vi "Read Ports_modified.vi"(0 "Refnum in":refnum<k20>, 2 "timeout (ms)":i32=5000, 5 "All 4 Ports":bool, 9 "number of elements":u64, 11 "error in":errorcluster, 13 "Simulated Data":bool) -> (4 "Refnum out":refnum<k20>, 6 "Read Region References":refnum<data-value>[](array[refnum]), 8 "Errors":u32[](array[numeric]), 10 "Elements Remaining":u32, 14 "Data Valid":bool, 15 "error out":errorcluster)   [LabVIEW 2016]
doc: "This VI wraps and calls the appropriate FIFO read node to access the FIFO corresponding to the input <b>port</b>\n\n<B>Input Parameters</B>\n\n<B>Refnum in</B> Receives a reference to the FPGA from the previous VI.\n\n<B>timeout (ms)</B> The timeout to pass to the FIFO read node\n\n<B>port</B> Selects which physical port to read from.\n\n<B>number of elements</B> Specifies the number of FIFO elements to read during this call.\n\n<B>error in</B> describes error conditions that occur before this node runs. This input provides standard error in functionality.\n\n<B>Output Parameters</B>\n\n<B>Refnum out</B> passes a reference to the FPGA to the next VI.\n\n<B>Receive Waveform</B> The data read from the device will be written to this output\n\n<B>Waveform Size</B> Indicates the number of samples in the output waveform\n\n<B>Elements Remaining</B> Indicates the number of samples presently waiting in the FIFO after the read.\n\n<B>error out</B> contains error information. This output provides standard error out functionality."
uses:
  Base Bitfile Reference.ctl
  <vilib>/Utility/error.llb/Error Cluster From Error Code.vi
  <vilib>/rvi/errors/niLvFpgaAdjustHostInterfaceError.vi
  <vilib>/rvi/interface/nirviMethod/nirviMethod.xnode
  <vilib>/rvi/interface/nirviReadWriteControl/nirviReadWriteControl.xnode
  Aurora Stream (NI 6592R) (Host).lvlib
  <vilib>/rvi/errors/niLvFpgaMergeErrorWithErrorCode.vi
  NiFpgaLv.dll
  <vilib>/rvi/interface/Simulation/niFpgaSimulationCallBeginRW.vi
  <vilib>/FPGAPlugInAG/Dynamic/niLvFpga_AcquireReadRegionFifo_Dynamic.vi
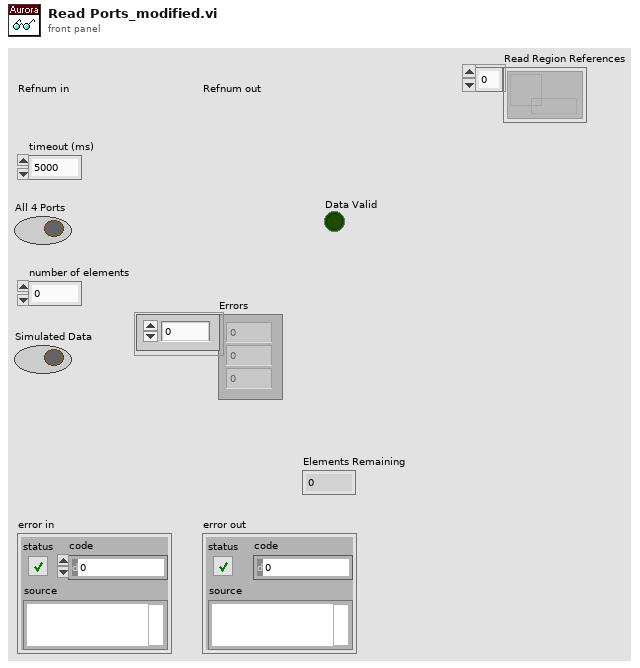
[diagram p1: front panel]
types:
  T1 = typedef "Aurora Stream (NI 6592R) (Host).lvlib/Base Bitfile Reference.ctl" = refnum<k20>
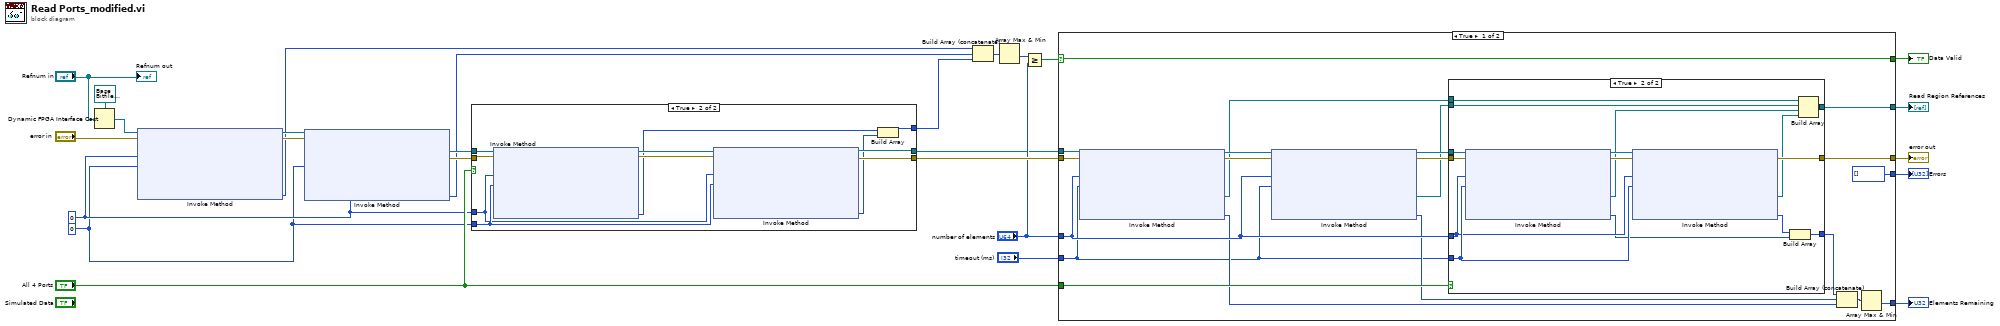
[diagram p0: block diagram]
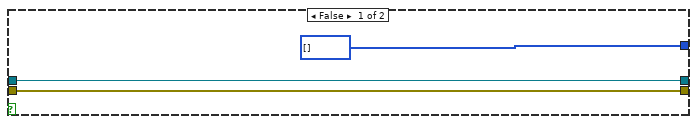
[diagram p2: hidden frame]
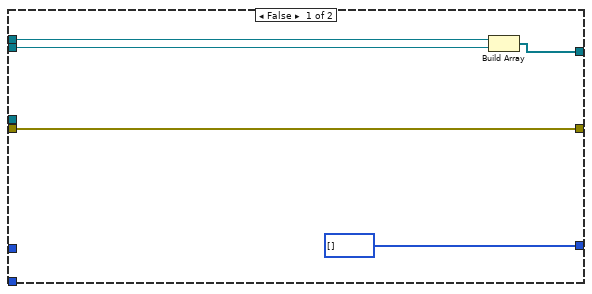
[diagram p3: hidden frame]
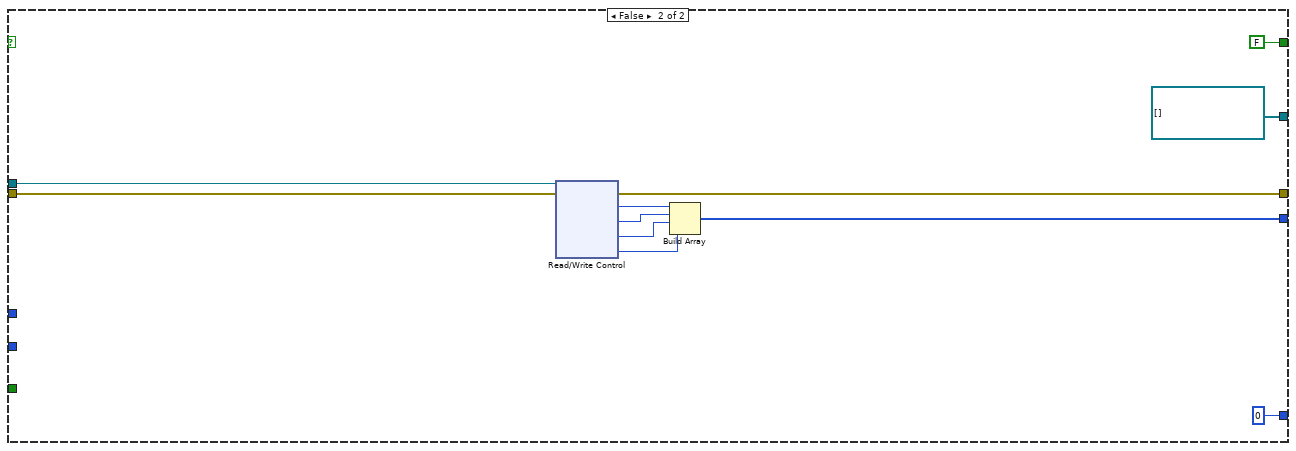
[diagram p4: hidden frame]
diagram:
  w5 = 0 ("Timeout (ms)")
  w6 = u32 0 ("Number of Elements")
  n1 = Dynamic FPGA Interface Cast(Session In=T1 refnum ("Aurora Sample Project"), Type="Refnum in") -> (Session Out=w13:T1)
  n2 = xnode "Invoke Method"("FPGA VI Reference In"=w13, "error in"="error in", "Number of Elements"=w6, "Timeout (ms)"=w5) -> ("FPGA VI Reference Out"=w11:T1, "error out"=w10:errorcluster, "Elements Remaining"=w2:u32)  [unwired: 2 out]
  n3 = xnode "Invoke Method"("FPGA VI Reference In"=w11, "error in"=w10, "Number of Elements"=w6, "Timeout (ms)"=w5) -> ("FPGA VI Reference Out"=w8:T1, "error out"=w9:errorcluster, "Elements Remaining"=w1:u32)  [unwired: 2 out]
  n4 = case shown="True" "All 4 Ports" {
    tunnel: w9 -> [w27 w38]
    tunnel: [w27 w35] -> w19
    tunnel: [u32[] [] w34] -> w22
    tunnel: w8 -> [w28 w37]
    tunnel: [w28 w36] -> w7
    tunnel: w6 -> [_ w30]
    tunnel: w5 -> [_ w31]
    frame False {
    }
    frame True {
      n5 = xnode "Invoke Method"("FPGA VI Reference In"=w37, "error in"=w38, "Number of Elements"=w30, "Timeout (ms)"=w31) -> ("FPGA VI Reference Out"=w39:T1, "error out"=w40:errorcluster, "Elements Remaining"=w33:u32)  [unwired: 2 out]
      n6 = xnode "Invoke Method"("FPGA VI Reference In"=w39, "error in"=w40, "Number of Elements"=w30, "Timeout (ms)"=w31) -> ("FPGA VI Reference Out"=w36:T1, "error out"=w35:errorcluster, "Elements Remaining"=w32:u32)  [unwired: 2 out]
      n7 = Build Array(w33, w32) -> (w34:u32[])
    }
  }
  n8 = Build Array (concatenate)(w2, w1, w22) -> (w21:u32[])
  n9 = Array Max & Min(array=w21) -> (min value=w20:u32)  [unwired: 3 out]
  n10 = Greater Or Equal?(x=w20, y="number of elements") -> (x >= y?=w18:bool)
  n11 = case shown="True" w18 {
    selector: w18 -> [w47 _]
    tunnel: [w54 w89] -> w26
    tunnel: "timeout (ms)" -> [w44 _]
    tunnel: w19 -> [w60 w90]
    tunnel: "number of elements" -> [w55 _]
    tunnel: "All 4 Ports" -> [w50 _]
    tunnel: [w51 u32 0] -> w15
    tunnel: [w41 refnum<data-value>[] []] -> w3
    tunnel: [u32[] [] w84] -> w14
    tunnel: w7 -> [w48 w83]
    tunnel: [w47 FALSE] -> w4
    frame True {
      n12 = xnode "Invoke Method"("FPGA VI Reference In"=w48, "error in"=w60, "Number of Elements"=w55, "Timeout (ms)"=w44) -> ("FPGA VI Reference Out"=w58:T1, "error out"=w59:errorcluster, "Read Region Reference"=w42:refnum<data-value>, "Elements Remaining"=w45:u32)  [unwired: 1 out]
      n13 = xnode "Invoke Method"("FPGA VI Reference In"=w58, "error in"=w59, "Number of Elements"=w55, "Timeout (ms)"=w44) -> ("FPGA VI Reference Out"=w56:T1, "error out"=w57:errorcluster, "Read Region Reference"=w43:refnum<data-value>, "Elements Remaining"=w46:u32)  [unwired: 1 out]
      n14 = case shown="True" w50 {
        tunnel: w57 -> [w65 w78]
        tunnel: w56 -> [_ w77]
        tunnel: w44 -> [_ w76]
        tunnel: w55 -> [_ w75]
        tunnel: [w65 w74] -> w54
        tunnel: [u32[] [] w73] -> w52
        tunnel: w43 -> [w62 w67]
        tunnel: w42 -> [w63 w70]
        tunnel: [w61 w66] -> w41
        frame False {
          n15 = Build Array(w63, w62) -> (w61:refnum<data-value>[])
        }
        frame True {
          n16 = xnode "Invoke Method"("FPGA VI Reference In"=w77, "error in"=w78, "Number of Elements"=w75, "Timeout (ms)"=w76) -> ("FPGA VI Reference Out"=w80:T1, "error out"=w79:errorcluster, "Read Region Reference"=w69:refnum<data-value>, "Elements Remaining"=w71:u32)  [unwired: 1 out]
          n17 = xnode "Invoke Method"("FPGA VI Reference In"=w80, "error in"=w79, "Number of Elements"=w75, "Timeout (ms)"=w76) -> ("error out"=w74:errorcluster, "Read Region Reference"=w68:refnum<data-value>, "Elements Remaining"=w72:u32)  [unwired: 2 out]
          n18 = Build Array(w72, w71) -> (w73:u32[])
          n19 = Build Array(w70, w67, w69, w68) -> (w66:refnum<data-value>[])
        }
      }
      n20 = Build Array (concatenate)(w52, w46, w45) -> (w53:u32[])
      n21 = Array Max & Min(array=w53) -> (min value=w51:u32)  [unwired: 3 out]
    }
    frame False {
      n22 = xnode "Read/Write Control"("FPGA VI Reference In"=w83, "error in"=w90) -> ("error out"=w89:errorcluster, "Er.Port 0"=w88:u32, "Er.Port 1"=w87:u32, "Er.Port 2"=w86:u32, "Er.Port 3"=w85:u32)  [unwired: 1 out]
      n23 = Build Array(w88, w87, w86, w85) -> (w84:u32[])
    }
  }
  "error out" <- w26
  "Elements Remaining" <- w15
  "Errors" <- w14
  "Data Valid" <- w4
  "Read Region References" <- w3
  "Refnum out" <- "Refnum in"
